vi "StartXYAlignmentAbsMove.vi"(8 "error in (no error)":errorcluster, 9 "X, Y mm":dbl[](array[numeric]), 11 "VXMMotionManager in":refnum<class "VXMMotionManager.lvclass">) -> (0 "error out":errorcluster, 3 "VXMMotionManager out":refnum<class "VXMMotionManager.lvclass">)   [LabVIEW 2019, in "VXMMotionManager.lvclass"]
doc: "Load up X position and Y position and go to the start and move case.\n\n**CAUTION** This absolute move does not move the probe up and out of the way.\n It moves in X and Y only in order s[eed up the alignment. \n Also, the alignment should be performed at a high Z position."
uses:
  VXMMotionManager.lvclass
  MoveAllAbsoluteStates.ctl
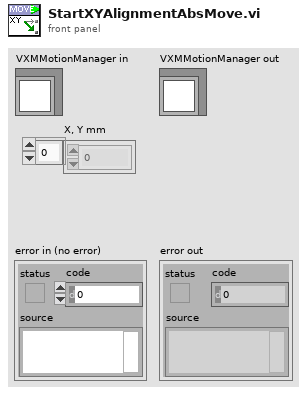
[diagram p1: front panel]
types:
  T1 = typedef "VXMMotionManager.lvclass/MoveAllAbsoluteStates.ctl" = enum16{"start next move", "wait motion end"}
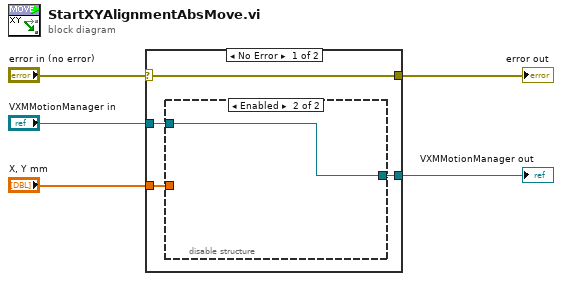
[diagram p0: block diagram]
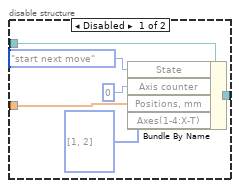
[diagram p2: hidden frame]
diagram:
  n1 = case shown="No Error" "error in (no error)" {
    selector: "error in (no error)" -> [w9 w18]
    tunnel: [w9 w18] -> w2
    tunnel: [w8 w17] -> w3
    tunnel: "VXMMotionManager in" -> [w7 w17]
    tunnel: "X, Y mm" -> [w6 _]
    frame No Error {
      n2 = disable-structure shown="Enabled" {
        disable-tunnel: [w14 w16] -> w8
        disable-tunnel: w7 -> [w12 w16]
        disable-tunnel: w6 -> [w11 _]
        frame Disabled {
          n3 = Bundle By Name(cluster=w12, "State"=MoveAllAbsoluteStates."start next move", "Axis counter"=0 ("Axis (0-3)"), "Positions, mm"=w11, "Axes(1-4:X-T)"=i32[] [1, 2] ("Axes(1-4:X-R)")) -> (w14:refnum<class "VXMMotionManager.lvclass">)
        }
        frame Enabled {
        }
      }
    }
    frame Error {
    }
  }
  "error out" <- w2
  "VXMMotionManager out" <- w3
